vi "Display Settings.vi"(11 "ConfigurationThisComponent in":refnum<class "Settings.lvclass">) -> (3 "ConfigurationThisComponent out":refnum<class "Settings.lvclass">)   [LabVIEW 2016, in "Settings.lvclass"]
uses:
  Settings.lvclass
  Typedefs/SerialSettings.ctl
  Typedefs/LogPath.ctl
  Typedefs/ConnectionSettings.ctl
  common_rt_hpilc/DataTypes/HPSettings.ctl
  common_rt_ilc/DataTypes/ILCSettings.ctl
  Typedefs/HPMT_Typedefs.lvlib
  common_rt_ilc/RTILC.lvlib
  common_rt_hpilc/RTHPILC.lvlib
panel:
  in  "ctrlRefArrayUsrEvnt":refnum<user-event>
  in  "ConfigTab":T1(tab)
  in  "Log Path":T2
  in  "ILC Serial Settings":T3={"Baud Rate"=921600, "Data Bits"=8, "Parity"=enum."None", "Flow Control"=0, "Stop Bits"=10, "Timeout (ms)"=2000, "Byte Count"=256, "Enable Termination Character"=FALSE, "Termination Char"=200} {"Termination Char" format="%x"; "Stop Bits" items=["1.0"=10, "1.5"=15, "2.0"=20]; "Flow Control" items=["None", "XON/XOFF", "RTS/CTS", "XON/XOFF & RTS/CTS", "DTR/DSR", "XON/XOFF & DTR/DSR"]; "Data Bits" min=5 max=8 step=1}
  in  "Displacement Serial Settings":T3={"Baud Rate"=921600, "Data Bits"=8, "Parity"=enum."None", "Flow Control"=0, "Stop Bits"=10, "Timeout (ms)"=2000, "Byte Count"=256, "Enable Termination Character"=FALSE, "Termination Char"=200} {"Termination Char" format="%x"; "Stop Bits" items=["1.0"=10, "1.5"=15, "2.0"=20]; "Flow Control" items=["None", "XON/XOFF", "RTS/CTS", "XON/XOFF & RTS/CTS", "DTR/DSR", "XON/XOFF & DTR/DSR"]; "Data Bits" min=5 max=8 step=1}
  in  "Connection Settings":T4
  in  "HPSettings":T5
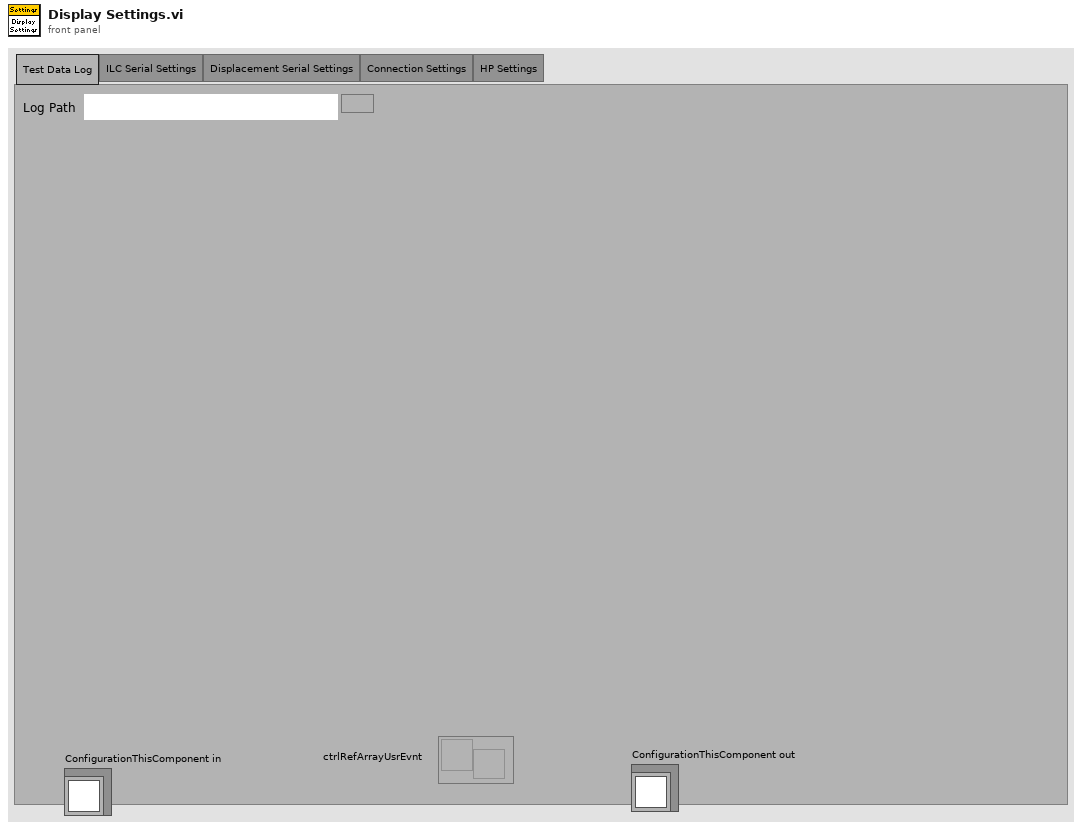
[diagram p1: front panel]
types:
  T1 = enum32{"Test Data Log", "ILC Serial Settings", "Displacement Serial Settings", "Connection Settings", "HP Settings"}
  T2 = typedef "HPMT_Typedefs.lvlib/LogPath.ctl" = path
  T3 = typedef "HPMT_Typedefs.lvlib/SerialSettings.ctl" = cluster{"Baud Rate":u32, "Data Bits":u16, "Parity":enum16{"None", "Odd", "Even", "Mark", "Space"}, "Flow Control":u16, "Stop Bits":u16, "Timeout (ms)":u32, "Byte Count":u32, "Enable Termination Character":bool, "Termination Char":u8}
  T4 = typedef "HPMT_Typedefs.lvlib/ConnectionSettings.ctl" = cluster{"ILC Port":refnum<visa-resource-name>, "Displacment Port\n":refnum<visa-resource-name>}
  T5 = typedef "RTHPILC.lvlib/HPSettings.ctl" = cluster{"ILCSettings":T6, "ID":i16, "ReferencePosition":i32}
  T6 = typedef "RTILC.lvlib/ILCSettings.ctl" = cluster{"Subnet":u8, "Address":u8}
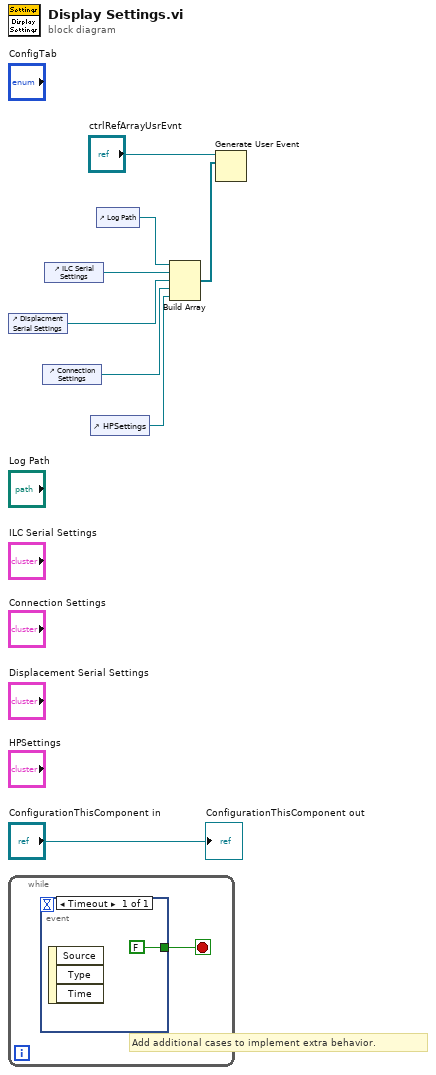
[diagram p0: block diagram]
diagram:
  n1 = control-ref of="Displacment Serial Settings"() -> (w1:refnum<vi>)
  n2 = while {
    stop <- w9 stop-if-true
    # "Add additional cases to implement extra behavior."
    n3 = event shown="[0] Timeout" {
      selector: _ -> [_]
      dyn-events: _ -> [_]
      timeout: _ -> [_]
      tunnel: [FALSE] -> w9
      event Timeout {
        n4 = event-data() -> ()  [unwired: 1 in, 3 out]
      }
    }
  }
  n5 = control-ref of="Connection Settings"() -> (w3:refnum<vi>)
  n6 = control-ref of="ILC Serial Settings"() -> (w4:refnum<vi>)
  n7 = control-ref of="HPSettings"() -> (w2:refnum<vi>)
  n8 = control-ref of="Log Path"() -> (w5:refnum<vi>)
  n9 = Build Array(w5, w4, w1, w3, w2) -> (w6:refnum<vi>[])
  n10 = Generate User Event(user event="ctrlRefArrayUsrEvnt", event data cluster=w6) -> ()  [unwired: 2 in, 2 out]
  "ConfigurationThisComponent out" <- "ConfigurationThisComponent in"
